vi "Apply CCD monitor Config Obj.vi"(8 "error in (no error)":errorcluster, 10 "Hardware.lvlib:CCD.lvlib:CCD Configuration.lvclass":refnum<class "CCD Configuration.lvclass">, 11 "Hardware.lvlib:CCD monitor.lvlib:CCD monitor configuration.lvclass":refnum<class "CCD monitor configuration.lvclass">) -> (0 "error out":errorcluster, 3 "Hardware.lvlib:CCD monitor.lvlib:CCD monitor configuration.lvclass 2":refnum<class "CCD monitor configuration.lvclass">)   [LabVIEW 2016, in "CCD monitor.lvlib" / "CCD monitor configuration.lvclass"]
uses:
  <userlib>/Common Components/Hardware/Abstract System/Monitor/CCD monitor configuration.lvclass
  <userlib>/Common Components/Hardware/CCD/CCD Configuration.lvclass
  <userlib>/Common Components/Hardware/Abstract System/Monitor/CCD monitor configuration.lvclass/CCD monitor configuration.ctl
  <userlib>/Common Components/Hardware/CCD/CCD Configuration.lvclass/CCD Configuration.ctl
  <userlib>/Common Components/Hardware/Abstract System/Monitor/CCD monitor.lvclass/CCD monitor.ctl
  <userlib>/Common Components/Hardware/Abstract Hardware/Hardware.lvclass/Hardware.ctl
  <userlib>/Common Components/Hardware/Abstract Hardware/Read Label.vi
  <userlib>/Common Components/Hardware/CCD/CCD/CCD.lvclass
  C:/Program Files (x86)/National Instruments/LabVIEW 2016/user.lib/Common Components/Hardware/Abstract Hardware/Hardware.lvclass
  <userlib>/Common Components/Hardware/Abstract System/Monitor/CCD monitor.lvclass
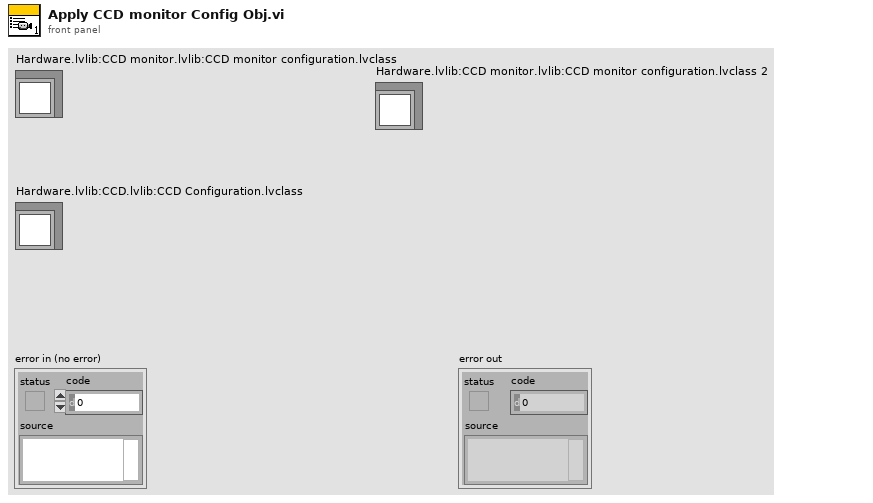
[diagram p1: front panel]
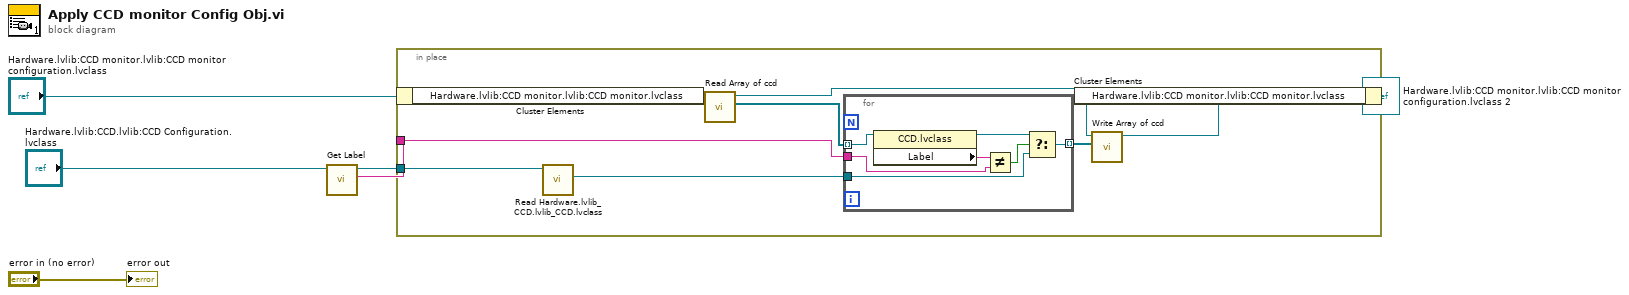
[diagram p0: block diagram]
diagram:
  n1 = call <userlib>:"Get Label.vi"("Hardware.lvlib:CCD.lvlib:CCD Configuration.lvclass"="Hardware.lvlib:CCD.lvlib:CCD Configuration.lvclass") -> ("Label"=w2:string, "Hardware.lvlib:CCD.lvlib:CCD Configuration.lvclass 2"=w3:refnum<class "CCD Configuration.lvclass">)  [unwired: 8 in, 1 out]
  n2 = in-place {
    in-place-border: w3 -> [w12]
    in-place-border: w2 -> [w10]
    n3 = in-place-cluster #1("Hardware.lvlib:CCD monitor.lvlib:CCD monitor configuration.lvclass") -> ("Hardware.lvlib:CCD monitor.lvlib:CCD monitor.lvclass"=w14:refnum<class "CCD monitor.lvclass">)
    n4 = call <userlib>:"Read Hardware.lvlib_CCD.lvlib_CCD.lvclass.vi"("CCD Configuration in"=w12) -> ("Hardware.lvlib:CCD.lvlib:CCD.lvclass"=w9:refnum<class "CCD.lvclass">)  [unwired: 8 in, 2 out]
    n5 = call <userlib>:"Read Array of ccd.vi"("CCD monitor in"=w14) -> ("Array of ccd"=w11:refnum<class "CCD.lvclass">[], "CCD monitor out"=w13:refnum<class "CCD monitor.lvclass">)  [unwired: 9 in]
    n6 = for {
      tunnel: w11 -> [w21] mode=indexing
      tunnel: w10 -> [w20]
      tunnel: w9 -> [w17]
      tunnel: [w16] -> w8 mode=indexing
      n7 = property class="CCD.lvclass"(reference=w21) -> (reference out=w18:refnum<class "CCD.lvclass">, "Label"=w15:string)  [unwired: 1 in, 1 out]
      n8 = Not Equal?(x=w15, y=w20) -> (x != y?=w19:bool)
      n9 = Select(t=w18, s=w19, f=w17) -> (s? t:f=w16:refnum<class "CCD.lvclass">)
    }
    n10 = call <userlib>:"Write Array of ccd.vi"("Array of ccd"=w8, "CCD monitor in"=w13) -> ("CCD monitor out"=w7:refnum<class "CCD monitor.lvclass">)  [unwired: 9 in]
    n11 = in-place-cluster #1("Hardware.lvlib:CCD monitor.lvlib:CCD monitor.lvclass"=w7) -> (→"Hardware.lvlib:CCD monitor.lvlib:CCD monitor configuration.lvclass 2":refnum<class "CCD monitor configuration.lvclass">)
  }
  "error out" <- "error in (no error)"
